vi "加载冷却系统控制.vi"(8 "error in (no error)":errorcluster caption="错误输入（无错误）") -> (0 "error out":errorcluster caption="错误输出")   [LabVIEW 2014]
doc: "该模板用于创建子VI。"
uses:
  glb/glb_data.vi
  <vilib>/Utility/config.llb/NI_LVConfig.lvlib
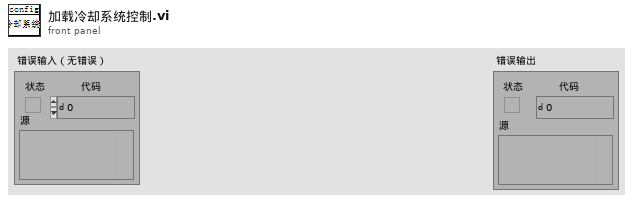
[diagram p1: front panel]
types:
  T1 = typedef "NI_LVConfig.lvlib/Config Data RefNum.ctl" = refnum<k1>
  T2 = cluster{"名称":string, "简称":string, "单位":string, "附加":string[], "类型":enum16{"测试模块", "FPGA", "cRIO", "其他设备", "总体展示"}}
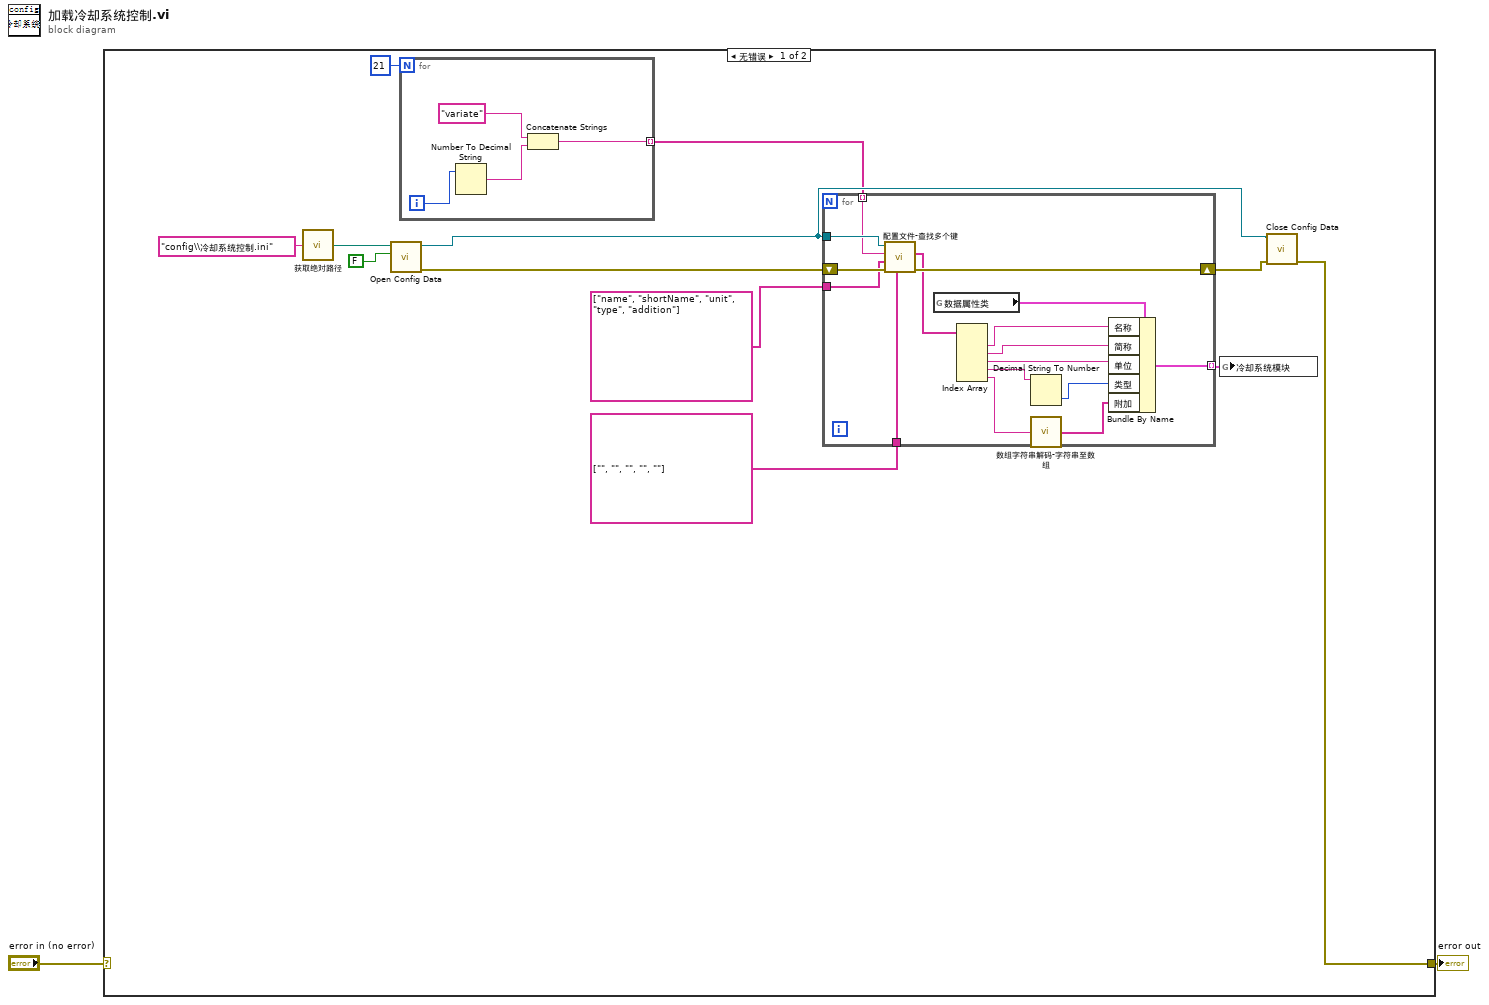
[diagram p0: block diagram]
diagram:
  n1 = case shown="无错误" "error in (no error)" {
    selector: "error in (no error)" -> [_ w35]
    tunnel: [w7 w35] -> w1
    frame No Error {
      n2 = call "获取绝对路径.vi"("relativePath"="config\\冷却系统控制.ini") -> ("absolutePath"=w13:path)
      n3 = call <vilib>:"Open Config Data.vi"("create file if necessary (T)"=FALSE, "configuration file path"=w13) -> ("error out"=w5:errorcluster, "refnum"=w8:T1)  [unwired: 7 in, 1 out]
      n4 = for {
        N: 21 -> [_]
        tunnel: [w15] -> w3 mode=indexing
        i -> [w18]
        n5 = Number To Decimal String(number=w18) -> (decimal integer string=w16:string)  [unwired: 1 in]
        n6 = Concatenate Strings("variate", w16) -> (w15:string)
      }
      n7 = for {
        tunnel: w8 -> [w33]
        tunnel: w3 -> [w32] mode=indexing
        tunnel: string[] ["name", "shortName", "unit", "type", "addition"] -> [w31]
        tunnel: string[] ["", "", "", "", ""] -> [w30]
        shift-right: [w29] -> w9
        shift-left: w5 -> [w34]
        tunnel: [w19] -> w6 mode=indexing
        n8 = call "配置文件-查找多个键.vi"("默认值"=w30, "错误输入（无错误）"=w34, "键名"=w31, "章名"=w32, "引用句柄输入"=w33) -> ("错误输出"=w29:errorcluster, "查询结果"=w20:string[])  [unwired: 4 in, 1 out]
        n9 = global read "类信息.vi" "数据属性类"() -> (w28:T2)
        n10 = Index Array(array=w20) -> (element #1=w27:string, element #2=w26:string, element #3=w25:string, element #4=w24:string, element #5=w22:string)  [unwired: 5 in]
        n11 = Decimal String To Number(string=w24) -> (number=w23:i32)  [unwired: 2 in, 1 out]
        n12 = call "数组字符串解码-字符串至数组.vi"("字符串"=w22) -> ("数组"=w21:string[])  [unwired: 1 in]
        n13 = Bundle By Name(cluster=w28, "名称"=w27, "简称"=w26, "单位"=w25, "类型"=w23, "附加"=w21) -> (w19:T2)
      }
      n14 = global write "glb_data.vi" "冷却系统模块"(w6) -> ()
      n15 = call <vilib>:"Close Config Data.vi"("error in (no error)"=w9, "refnum"=w8) -> ("error out"=w7:errorcluster)  [unwired: 8 in, 1 out]
    }
    frame Error {
    }
  }
  "error out" <- w1
